vi "Get Nb of Cars.vi"(8 "error in (no error)":errorcluster, 11 "CarPool in":refnum<class "CarPool.lvclass">) -> (0 "error out":errorcluster, 2 "Nb Cars":i32, 3 "CarPool out":refnum<class "CarPool.lvclass">)   [LabVIEW 2017, in "CarPool.lvclass"]
uses:
  CarPool.lvclass
  CarPool.lvclass/CarPool.ctl
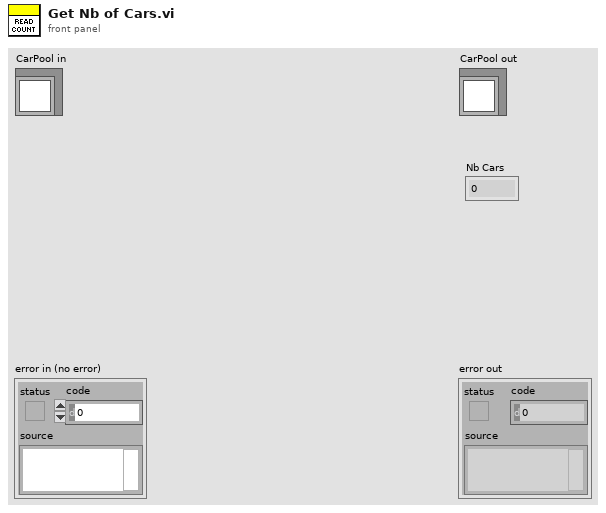
[diagram p1: front panel]
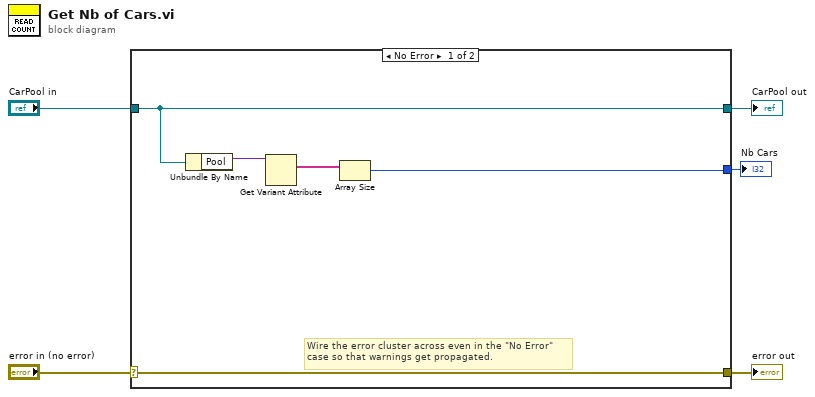
[diagram p0: block diagram]
diagram:
  n1 = case shown="No Error" "error in (no error)" {
    selector: "error in (no error)" -> [w10 w12]
    tunnel: [w10 w12] -> w4
    tunnel: [w9 w11] -> w2
    tunnel: "CarPool in" -> [w9 w11]
    tunnel: [w6 _] -> w1
    frame No Error {
      # "Wire the error cluster across even in the \"No Error\"\ncase so that warnings get propagated."
      n2 = Unbundle By Name(w9) -> ("Pool"=w8:variant)
      n3 = Get Variant Attribute(Variant=w8) -> (names=w7:string[])  [unwired: 3 in, 3 out]
      n4 = Array Size(array=w7) -> (size(s)=w6:i32)
    }
    frame Error {
    }
  }
  "error out" <- w4
  "CarPool out" <- w2
  "Nb Cars" <- w1
